vi "User Tags Tree.vi"   [LabVIEW 2013]
uses:
  <vilib>/UserTags/UserTags.lvlib
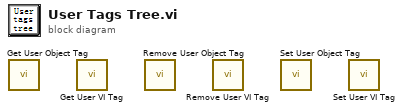
[diagram p0: block diagram]
diagram:
  n1 = call <vilib>:"Get User Object Tag.vi"() -> ()  [unwired: 8 in, 4 out]
  n2 = call <vilib>:"Get User VI Tag.vi"() -> ()  [unwired: 8 in, 4 out]
  n3 = call <vilib>:"Remove User Object Tag.vi"() -> ()  [unwired: 9 in, 3 out]
  n4 = call <vilib>:"Remove User VI Tag.vi"() -> ()  [unwired: 9 in, 3 out]
  n5 = call <vilib>:"Set User Object Tag.vi"() -> ()  [unwired: 9 in, 3 out]
  n6 = call <vilib>:"Set User VI Tag.vi"() -> ()  [unwired: 9 in, 3 out]
